vi "修改密码-new.vi"() -> ()   [LabVIEW 2015]
panel:
  in  "文件（使用对话框）":path=path "C:/Users/Administrator/Desktop/跳远项目上位机/登录界面/user.txt"
  in  "确定按钮":bool
  in  "新密码":string
  in  "新账号":string
  in  "密码":string
  in  "账号":string
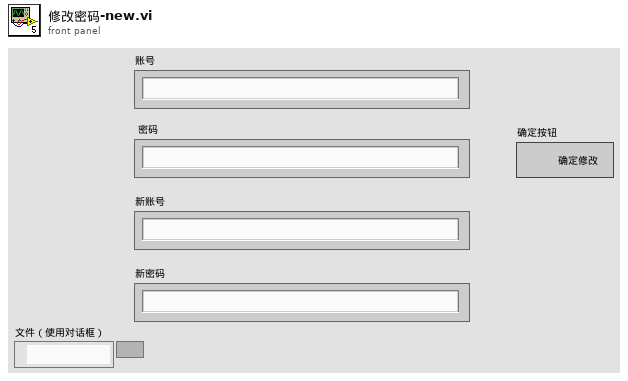
[diagram p1: front panel]
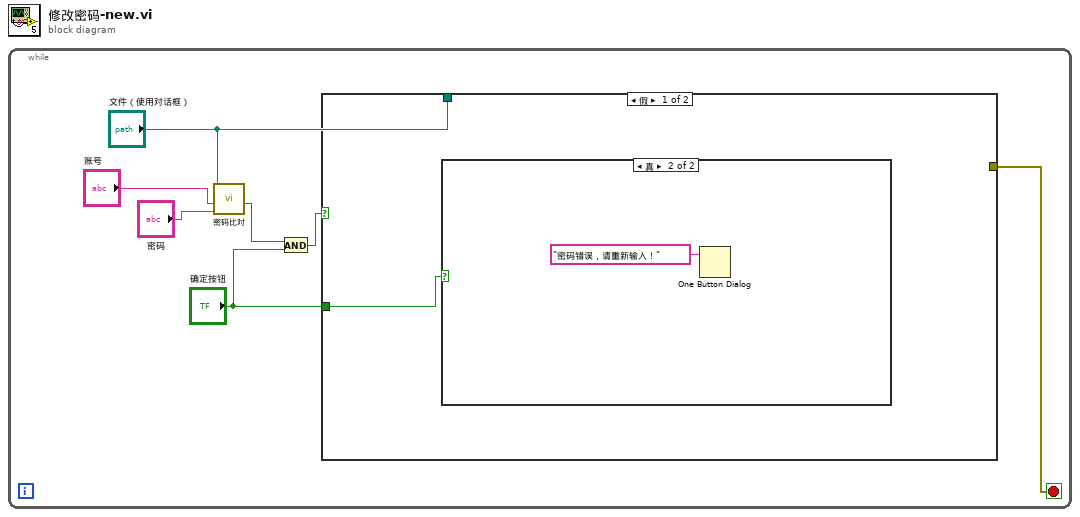
[diagram p0: block diagram]
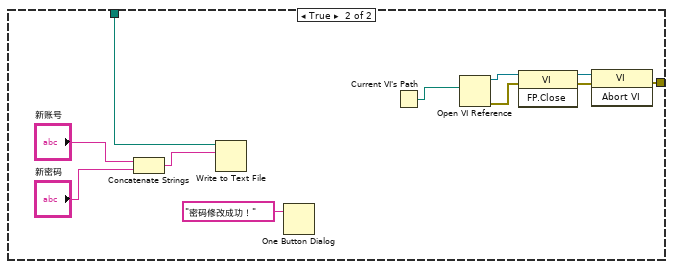
[diagram p3: hidden frame]
diagram:
  n1 = while {
    stop <- w2 stop-if-true
    n2 = call "密码比对.vi"("密码"="密码", "账户"="账号", "文件（使用对话框）"="文件（使用对话框）") -> ("x = y?"=w5:bool)  [unwired: 8 in]
    n3 = And(x=w5, y="确定按钮") -> (x .and. y?=w4:bool)
    n4 = case shown="假" w4 {
      tunnel: "文件（使用对话框）" -> [_ w17]
      tunnel: [_ w10] -> w2
      tunnel: "确定按钮" -> [w8 _]
      frame False {
        n5 = case shown="真" w8 {
          frame False {
          }
          frame True {
            n6 = One Button Dialog(message="密码错误，请重新输入！" ("消息")) -> ()  [unwired: 1 in, 1 out]
          }
        }
      }
      frame True {
        n7 = Concatenate Strings("新账号", "新密码") -> (w18:string)
        n8 = Write to Text File(file (use dialog)=w17, text=w18) -> ()  [unwired: 2 in, 3 out]
        n9 = One Button Dialog(message="密码修改成功！" ("消息")) -> ()  [unwired: 1 in, 1 out]
        n10 = Current VI's Path() -> (path=w15:path)
        n11 = Open VI Reference(vi path=w15) -> (vi reference=w14:refnum<vi>, error out=w13:errorcluster)  [unwired: 5 in]
        n12 = invoke class="VI" method="FP.Close"(reference=w14, error in=w13) -> (reference out=w12:refnum<vi>, error out=w11:errorcluster)  [unwired: 1 in, 1 out]
        n13 = invoke class="VI" method="Abort VI"(reference=w12, error in=w11) -> (error out=w10:errorcluster)  [unwired: 1 in, 2 out]
      }
    }
  }
